vi "start.vi"(8 "error in (no error)":errorcluster, 10 "Reference Voltage Vref":dbl[unit] min=-10.0 max=10.0 format="%.3f", 11 "ForceSensor in":refnum<class "ForceSensor.lvclass">) -> (0 "error out":errorcluster, 3 "ForceSensor out":refnum<class "ForceSensor.lvclass">)   [LabVIEW 2013, in "ForceSensor.lvclass"]
uses:
  ForceSensor.lvclass
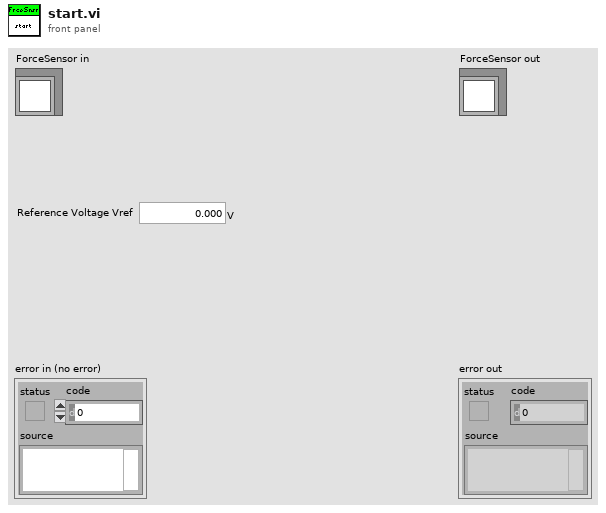
[diagram p1: front panel]
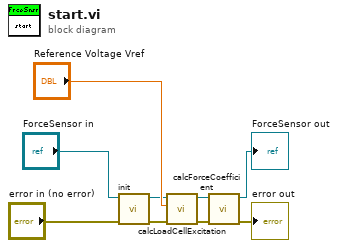
[diagram p0: block diagram]
diagram:
  n1 = call "init.vi"("error in (no error)"="error in (no error)", "ForceSensor in"="ForceSensor in") -> ("error out"=w4:errorcluster, "ForceSensor out"=w8:refnum<class "ForceSensor.lvclass">)  [unwired: 8 in]
  n2 = call "calcLoadCellExcitation.vi"("error in (no error)"=w4, "Reference Voltage Vref"="Reference Voltage Vref", "ForceSensor in"=w8) -> ("error out"=w3:errorcluster, "ForceSensor out"=w7:refnum<class "ForceSensor.lvclass">)  [unwired: 7 in]
  n3 = call "calcForceCoefficient.vi"("error in (no error)"=w3, "ForceSensor in"=w7) -> ("error out"=→"error out":errorcluster, "ForceSensor out"=→"ForceSensor out":refnum<class "ForceSensor.lvclass">)  [unwired: 8 in]
